vi "HTTPS Client Test.vi"() -> ()   [LabVIEW 2013]
uses:
  NI OpenSSL Socket/SSL_Lib/SSL/X509_Verify_Result.ctl
  NI OpenSSL Socket/SSL_Lib/SSL-Lib/Library Paths.ctl
  NI OpenSSL Socket/SSL_Lib/SSL-Context/SSL Options.ctl
  NI OpenSSL Socket/SSL_Lib/SSL/SSL_Mode.ctl
  NI OpenSSL Socket/SSL_Lib/SSL-Context/SSL Verify Mode.ctl
  NI OpenSSL Socket/SSL_Lib/SSL/X509_Host_Verify_Flags.ctl
  NI OpenSSL Socket/SSL_Lib/SSL-Lib/SSL-Lib.lvclass
  NI OpenSSL Socket/SSL_Lib/SSL-Context/SSL-Context.lvclass
  NI OpenSSL Socket/SSL_Lib/BIO/BIO.lvclass
  NI OpenSSL Socket/SSL_Lib/SSL/SSL.lvclass
  NI OpenSSL Socket/SSL_Lib/X509-Cert/X509-Cert.lvclass
panel:
  out "verify result":T1
  out "issuer name":string
  out "subject name":string
  out "String read":string
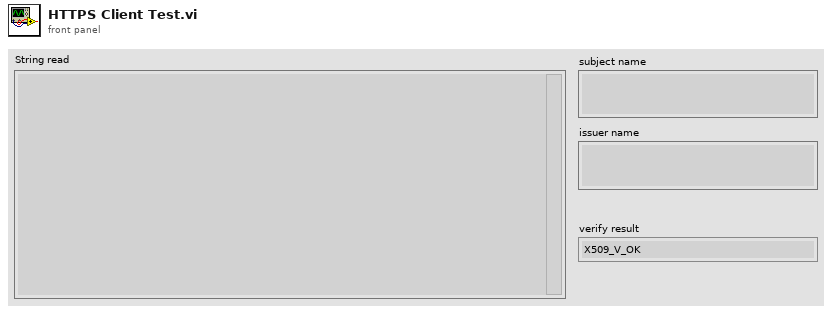
[diagram p1: front panel]
types:
  T1 = typedef "OpenSSL Socket.lvlib/SSL.lvclass/X509_Verify_Result.ctl" = enum16{"X509_V_OK", "X509_V_ERR_UNSPECIFIED", "X509_V_ERR_UNABLE_TO_GET_ISSUER_CERT", "X509_V_ERR_UNABLE_TO_GET_CRL", "X509_V_ERR_UNABLE_TO_DECRYPT_CERT_SIGNATURE", "X509_V_ERR_UNABLE_TO_DECRYPT_CRL_SIGNATURE", "X509_V_ERR_UNABLE_TO_DECODE_ISSUER_PUBLIC_KEY", "X509_V_ERR_CERT_SIGNATURE_FAILURE", "X509_V_ERR_CRL_SIGNATURE_FAILURE", "X509_V_ERR_CERT_NOT_YET_VALID", "X509_V_ERR_CERT_HAS_EXPIRED", "X509_V_ERR_CRL_NOT_YET_VALID", "X509_V_ERR_CRL_HAS_EXPIRED", "X509_V_ERR_ERROR_IN_CERT_NOT_BEFORE_FIELD", "X509_V_ERR_ERROR_IN_CERT_NOT_AFTER_FIELD", "X509_V_ERR_ERROR_IN_CRL_LAST_UPDATE_FIELD", "X509_V_ERR_ERROR_IN_CRL_NEXT_UPDATE_FIELD", "X509_V_ERR_OUT_OF_MEM", "X509_V_ERR_DEPTH_ZERO_SELF_SIGNED_CERT", "X509_V_ERR_SELF_SIGNED_CERT_IN_CHAIN", "X509_V_ERR_UNABLE_TO_GET_ISSUER_CERT_LOCALLY", "X509_V_ERR_UNABLE_TO_VERIFY_LEAF_SIGNATURE", "X509_V_ERR_CERT_CHAIN_TOO_LONG", "X509_V_ERR_CERT_REVOKED", "X509_V_ERR_INVALID_CA", "X509_V_ERR_PATH_LENGTH_EXCEEDED", "X509_V_ERR_INVALID_PURPOSE", "X509_V_ERR_CERT_UNTRUSTED", "X509_V_ERR_CERT_REJECTED", "X509_V_ERR_SUBJECT_ISSUER_MISMATCH", "X509_V_ERR_AKID_SKID_MISMATCH", "X509_V_ERR_AKID_ISSUER_SERIAL_MISMATCH", "X509_V_ERR_KEYUSAGE_NO_CERTSIGN", "X509_V_ERR_UNABLE_TO_GET_CRL_ISSUER", "X509_V_ERR_UNHANDLED_CRITICAL_EXTENSION", "X509_V_ERR_KEYUSAGE_NO_CRL_SIGN", "X509_V_ERR_UNHANDLED_CRITICAL_CRL_EXTENSION", "X509_V_ERR_INVALID_NON_CA", "X509_V_ERR_PROXY_PATH_LENGTH_EXCEEDED", "X509_V_ERR_KEYUSAGE_NO_DIGITAL_SIGNATURE", "X509_V_ERR_PROXY_CERTIFICATES_NOT_ALLOWED", "X509_V_ERR_INVALID_EXTENSION", "X509_V_ERR_INVALID_POLICY_EXTENSION", "X509_V_ERR_NO_EXPLICIT_POLICY", "X509_V_ERR_DIFFERENT_CRL_SCOPE", "X509_V_ERR_UNSUPPORTED_EXTENSION_FEATURE", "X509_V_ERR_UNNESTED_RESOURCE", "X509_V_ERR_PERMITTED_VIOLATION", "X509_V_ERR_EXCLUDED_VIOLATION", "X509_V_ERR_SUBTREE_MINMAX", "X509_V_ERR_APPLICATION_VERIFICATION", "X509_V_ERR_UNSUPPORTED_CONSTRAINT_TYPE", "X509_V_ERR_UNSUPPORTED_CONSTRAINT_SYNTAX", "X509_V_ERR_UNSUPPORTED_NAME_SYNTAX", "X509_V_ERR_CRL_PATH_VALIDATION_ERROR", "N/A", "X509_V_ERR_SUITE_B_INVALID_VERSION", "X509_V_ERR_SUITE_B_INVALID_ALGORITHM", "X509_V_ERR_SUITE_B_INVALID_CURVE", "X509_V_ERR_SUITE_B_INVALID_SIGNATURE_ALGORITHM", "X509_V_ERR_SUITE_B_LOS_NOT_ALLOWED", "X509_V_ERR_SUITE_B_CANNOT_SIGN_P_384_WITH_P_256", "X509_V_ERR_HOSTNAME_MISMATCH", "X509_V_ERR_EMAIL_MISMATCH", "X509_V_ERR_IP_ADDRESS_MISMATCH", "X509_V_ERR_INVALID_CALL", "X509_V_ERR_STORE_LOOKUP", "X509_V_ERR_PROXY_SUBJECT_NAME_VIOLATION"}
  T2 = typedef "OpenSSL Socket.lvlib/SSL.lvclass/SSL_Mode.ctl" = i32
  T3 = typedef "OpenSSL Socket.lvlib/SSL-Context.lvclass/SSL Options.ctl" = i32
  T4 = typedef "OpenSSL Socket.lvlib/SSL-Lib.lvclass/Library Paths.ctl" = cluster{"SSL Library Path":path, "Crypto Library Path":path}
  T5 = typedef "OpenSSL Socket.lvlib/SSL-Context.lvclass/SSL Verify Mode.ctl" = i32
  T6 = typedef "OpenSSL Socket.lvlib/SSL.lvclass/X509_Host_Verify_Flags.ctl" = u32
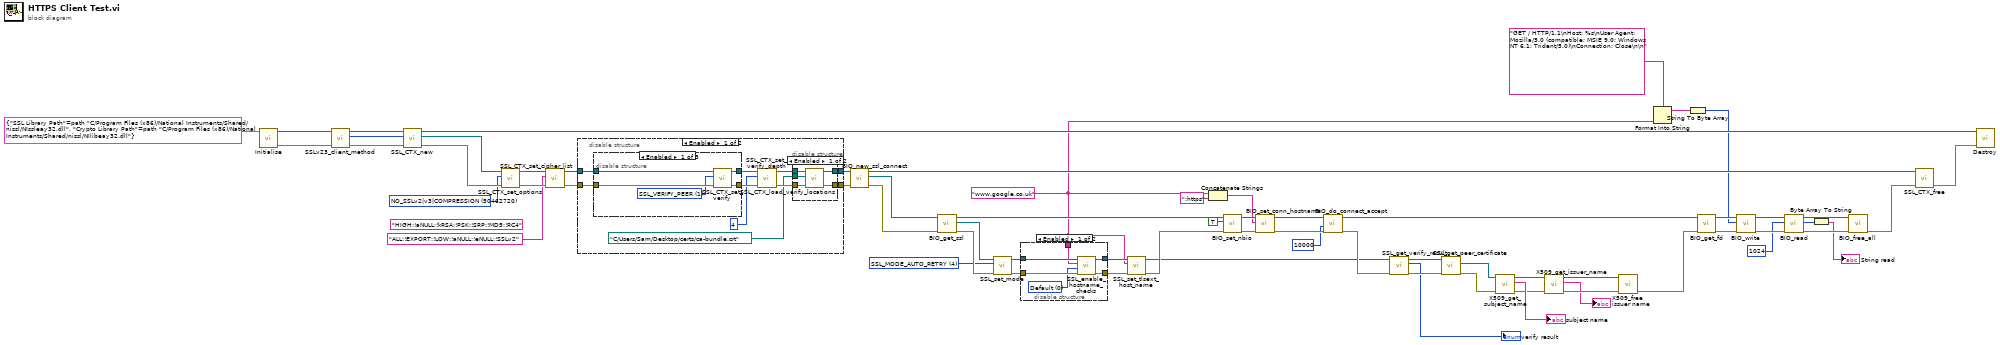
[diagram p0: block diagram]
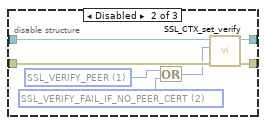
[diagram p3: hidden frame]
diagram:
  w6 = "www.google.co.uk" ("Hostname")
  (unwired) "HIGH:!aNULL:!kRSA:!PSK:!SRP:!MD5:!RC4" ("Cipher List")
  w36 = T2 4 items=["None"=0, "SSL_MODE_ENABLE_PARTIAL_WRITE"=1, "SSL_MODE_ACCEPT_MOVING_WRITE_BUFFER"=2, "SSL_MODE_AUTO_RETRY"=4, "SSL_MODE_RELEASE_BUFFERS"=16, "SSL_MODE_SEND_FALLBACK_SCSV"=128] ("Mode")
  w37 = T3 50462720 items=["None"=0, "NO_SSLv2|v3|COMPRESSION"=50462720, "SSL_OP_NO_COMPRESSION"=131072, "SSL_OP_NO_SSLv2"=16777216, "SSL_OP_NO_SSLv3"=33554432, "SSL_OP_NO_TLSv1"=67108864, "SSL_OP_NO_TLSv1_2"=134217728, "SSL_OP_NO_TLSv1_1"=268435456] ("Options")
  n1 = call "Initialise.vi"("Library Paths"=T4 {"SSL Library Path"=path "C:/Program Files (x86)/National Instruments/Shared/nissl/NIssleay32.dll", "Crypto Library Path"=path "C:/Program Files (x86)/National Instruments/Shared/nissl/NIlibeay32.dll"}) -> ("error out"=w63:errorcluster, "SSL-Lib out"=w67:refnum<class "SSL-Lib.lvclass">)  [unwired: 9 in]
  n2 = call "SSLv23_client_method.vi"("error in (no error)"=w63, "SSL-Lib in"=w67) -> ("error out"=w61:errorcluster, "*SSL_Method"=w66:u64, "SSL-Lib out"=w65:refnum<class "SSL-Lib.lvclass">)  [unwired: 7 in]
  n3 = call "SSL_CTX_new.vi"("error in (no error)"=w61, "*SSL_Method"=w66, "SSL-Lib in"=w65) -> ("error out"=w38:errorcluster, "SSL-Context out"=w39:refnum<class "SSL-Context.lvclass">, "SSL-Lib out"=w60:refnum<class "SSL-Lib.lvclass">)  [unwired: 6 in]
  n4 = call "SSL_CTX_set_options.vi"("error in (no error)"=w38, "Options"=w37, "SSL-Context in"=w39) -> ("error out"=w17:errorcluster, "SSL-Context out"=w20:refnum<class "SSL-Context.lvclass">)  [unwired: 7 in]
  n5 = call "SSL_CTX_set_cipher_list.vi"("error in (no error)"=w17, "Cipher List"="ALL:!EXPORT:!LOW:!aNULL:!eNULL:!SSLv2", "SSL-Context in"=w20) -> ("error out"=w18:errorcluster, "SSL-Context out"=w19:refnum<class "SSL-Context.lvclass">)  [unwired: 7 in]
  n6 = disable-structure shown="Enabled" {
    disable-tunnel: [w77 w100] -> w35
    disable-tunnel: [w76 w99] -> w34
    disable-tunnel: w19 -> [w75 w100]
    disable-tunnel: w18 -> [w74 w99]
    frame Enabled {
      n7 = disable-structure shown="Enabled" {
        disable-tunnel: w75 -> [w82 w89 w91]
        disable-tunnel: w74 -> [w81 w88 w90]
        disable-tunnel: [w80 w87 w90] -> w73
        disable-tunnel: [w79 w86 w91] -> w72
        frame Enabled {
          w78 = T5 1 items=["SSL_VERIFY_NONE"=0, "SSL_VERIFY_PEER"=1, "SSL_VERIFY_FAIL_IF_NO_PEER_CERT"=2, "SSL_VERIFY_CLIENT_ONCE"=4] ("Mode")
          n8 = call "SSL_CTX_set_verify.vi"("error in (no error)"=w81, "Mode"=w78, "SSL-Context in"=w82) -> ("error out"=w80:errorcluster, "SSL-Context out"=w79:refnum<class "SSL-Context.lvclass">)  [unwired: 7 in]
        }
        frame Disabled {
          w85 = T5 2 items=["SSL_VERIFY_NONE"=0, "SSL_VERIFY_PEER"=1, "SSL_VERIFY_FAIL_IF_NO_PEER_CERT"=2, "SSL_VERIFY_CLIENT_ONCE"=4] ("Mode")
          w84 = T5 1 items=["SSL_VERIFY_NONE"=0, "SSL_VERIFY_PEER"=1, "SSL_VERIFY_FAIL_IF_NO_PEER_CERT"=2, "SSL_VERIFY_CLIENT_ONCE"=4] ("Mode")
          n9 = Or(x=w84, y=w85) -> (x .or. y?=w83:T5)
          n10 = call "SSL_CTX_set_verify.vi"("error in (no error)"=w88, "Mode"=w83, "SSL-Context in"=w89) -> ("error out"=w87:errorcluster, "SSL-Context out"=w86:refnum<class "SSL-Context.lvclass">)  [unwired: 7 in]
        }
        frame Disabled {
        }
      }
      n11 = call "SSL_CTX_set_verify_depth.vi"("error in (no error)"=w73, "Depth"=4, "SSL-Context in"=w72) -> ("error out"=w69:errorcluster, "SSL-Context out"=w70:refnum<class "SSL-Context.lvclass">)  [unwired: 7 in]
      n12 = disable-structure shown="Enabled" {
        disable-tunnel: [w96 w98] -> w77
        disable-tunnel: [w95 w97] -> w76
        disable-tunnel: w70 -> [w94 w98]
        disable-tunnel: w69 -> [w93 w97]
        disable-tunnel: path "C:/Users/Sam/Desktop/certs/ca-bundle.crt" ("Path to CA bundle") -> [w92 _]
        frame Enabled {
          n13 = call "SSL_CTX_load_verify_locations.vi"("error in (no error)"=w93, "Path to CA bundle"=w92, "SSL-Context in"=w94) -> ("error out"=w95:errorcluster, "SSL-Context out"=w96:refnum<class "SSL-Context.lvclass">)  [unwired: 7 in]
        }
        frame Disabled {
        }
      }
    }
    frame Disabled {
    }
  }
  n14 = call "BIO_new_ssl_connect.vi"("error in (no error)"=w34, "SSL-Context in"=w35) -> ("error out"=w56:errorcluster, "BIO out"=w57:refnum<class "BIO.lvclass">, "SSL-Context out"=w59:refnum<class "SSL-Context.lvclass">)  [unwired: 7 in]
  n15 = call "BIO_get_ssl.vi"("error in (no error)"=w56, "BIO in"=w57) -> ("error out"=w54:errorcluster, "SSL out"=w55:refnum<class "SSL.lvclass">, "BIO out"=w47:refnum<class "BIO.lvclass">)  [unwired: 7 in]
  n16 = call "SSL_set_mode.vi"("error in (no error)"=w54, "Mode"=w36, "SSL in"=w55) -> ("error out"=w16:errorcluster, "SSL out"=w15:refnum<class "SSL.lvclass">)  [unwired: 7 in]
  n17 = disable-structure shown="Enabled" {
    disable-tunnel: w16 -> [w106 w107]
    disable-tunnel: w15 -> [w105 w108]
    disable-tunnel: [w104 w107] -> w9
    disable-tunnel: [w103 w108] -> w10
    disable-tunnel: w6 -> [w101 _]
    frame Enabled {
      w102 = T6 0 items=["Default"=0, "X509_CHECK_FLAG_ALWAYS_CHECK_SUBJECT"=1, "X509_CHECK_FLAG_NO_WILDCARDS"=2, "X509_CHECK_FLAG_NO_PARTIAL_WILDCARDS"=4, "X509_CHECK_FLAG_MULTI_LABEL_WILDCARDS"=8, "X509_CHECK_FLAG_SINGLE_LABEL_SUBDOMAINS"=16] ("Verification Flags")
      n18 = call "SSL_enable_hostname_checks.vi"("error in (no error)"=w106, "Verification Flags"=w102, "Hostname"=w101, "SSL in"=w105) -> ("error out"=w104:errorcluster, "SSL out"=w103:refnum<class "SSL.lvclass">)  [unwired: 6 in]
    }
    frame Disabled {
    }
  }
  n19 = call "SSL_set_tlsext_host_name.vi"("error in (no error)"=w9, "Hostname"=w6, "SSL in"=w10) -> ("error out"=w8:errorcluster, "SSL out"=w7:refnum<class "SSL.lvclass">)  [unwired: 7 in]
  n20 = Concatenate Strings(w6, ":https" ("string")) -> (w13:string)
  n21 = call "BIO_set_nbio.vi"("error in (no error)"=w8, "Non-Blocking?"=TRUE, "BIO in"=w47) -> ("error out"=w48:errorcluster, "BIO out"=w45:refnum<class "BIO.lvclass">)  [unwired: 7 in]
  n22 = call "BIO_set_conn_hostname.vi"("error in (no error)"=w48, "Hostname"=w13, "BIO in"=w45) -> ("error out"=w43:errorcluster, "BIO out"=w44:refnum<class "BIO.lvclass">)  [unwired: 7 in]
  n23 = call "BIO_do_connect_accept.vi"("error in (no error)"=w43, "Timeout (10000ms)"=u32 10000, "BIO in"=w44) -> ("error out"=w24:errorcluster, "BIO out"=w42:refnum<class "BIO.lvclass">)  [unwired: 7 in]
  n24 = call "SSL_get_verify_result.vi"("error in (no error)"=w24, "SSL-Lib in"=w7) -> ("error out"=w23:errorcluster, "verify result"=→"verify result":T1, "SSL-Lib out"=w22:refnum<class "SSL.lvclass">)  [unwired: 7 in]
  n25 = call "SSL_get_peer_certificate.vi"("error in (no error)"=w23, "SSL-Lib in"=w22) -> ("error out"=w31:errorcluster, "X509-Cert out"=w32:refnum<class "X509-Cert.lvclass">)  [unwired: 7 in, 1 out]
  n26 = call "X509_get_subject_name.vi"("error in (no error)"=w31, "X509-Cert in"=w32) -> ("error out"=w27:errorcluster, "subject name"=→"subject name":string, "X509-Cert out"=w29:refnum<class "X509-Cert.lvclass">)  [unwired: 7 in]
  n27 = call "X509_get_issuer_name.vi"("error in (no error)"=w27, "X509-Cert in"=w29) -> ("error out"=w26:errorcluster, "issuer name"=→"issuer name":string, "X509-Cert out"=w28:refnum<class "X509-Cert.lvclass">)  [unwired: 7 in]
  n28 = call "X509_free.vi"("error in (no error)"=w26, "X509-Cert in"=w28) -> ("error out"=w33:errorcluster)  [unwired: 9 in]
  n29 = Format Into String(format string="GET / HTTP/1.1\nHost: %s\nUser Agent: Mozilla/5.0 (compatible; MSIE 9.0; Windows NT 6.1; Trident/5.0)\nConnection: Close\n\n" ("String to write"), w6) -> (resulting string=w11:string)  [unwired: 2 in, 1 out]
  n30 = String To Byte Array(string=w11) -> (unsigned byte array=w5:u8[])
  n31 = call "BIO_get_fd.vi"("error in (no error)"=w33, "BIO in"=w42) -> ("error out"=w41:errorcluster, "BIO out"=w40:refnum<class "BIO.lvclass">)  [unwired: 7 in, 1 out]
  n32 = call "BIO_write.vi"("error in (no error)"=w41, "Bytes to write"=w5, "BIO in"=w40) -> ("error out"=w53:errorcluster, "BIO out"=w52:refnum<class "BIO.lvclass">)  [unwired: 6 in, 1 out]
  n33 = call "BIO_read.vi"("error in (no error)"=w53, "bytes to read"=1024, "BIO in"=w52) -> ("error out"=w49:errorcluster, "Bytes read"=w50:u8[], "BIO out"=w51:refnum<class "BIO.lvclass">)  [unwired: 6 in]
  n34 = Byte Array To String(unsigned byte array=w50) -> (string=→"String read":string)
  n35 = call "BIO_free_all.vi"("error in (no error)"=w49, "BIO in"=w51) -> ("error out"=w58:errorcluster)  [unwired: 9 in]
  n36 = call "SSL_CTX_free.vi"("error in (no error)"=w58, "SSL-Context in"=w59) -> ("error out"=w62:errorcluster)  [unwired: 9 in]
  n37 = call "Destroy.vi"("error in (no error)"=w62, "SSL-Lib in"=w60) -> ()  [unwired: 9 in, 1 out]
